vi "Init Channels.vi"(8 "error in (no error)":errorcluster, 11 "Device Item Ref In":T2 format="%.0x") -> (0 "error out":errorcluster, 1 "Output Refs":T1[](array[typedef]) format="%.0x", 2 "Output Values":dbl[](array[numeric]), 3 "Input Refs":T1[](array[typedef]) format="%.0x", 5 "Input Values":dbl[](array[numeric]))   [LabVIEW 2011, in "Interpolate 1D Array Custom Device.lvlib"]
uses:
  Interpolate 1D Array Custom Device.lvlib
  <vilib>/NI Veristand/Custom Device API/Custom Device Item Ref.ctl
  <vilib>/NI Veristand/Custom Device API/Data Reference.ctl
  <vilib>/NI Veristand/Custom Device API/Custom Device Channel Type.ctl
  <vilib>/NI Veristand/Custom Device API/Data Access Type.ctl
  <vilib>/NI Veristand/Custom Device API/Custom Device API.lvlib
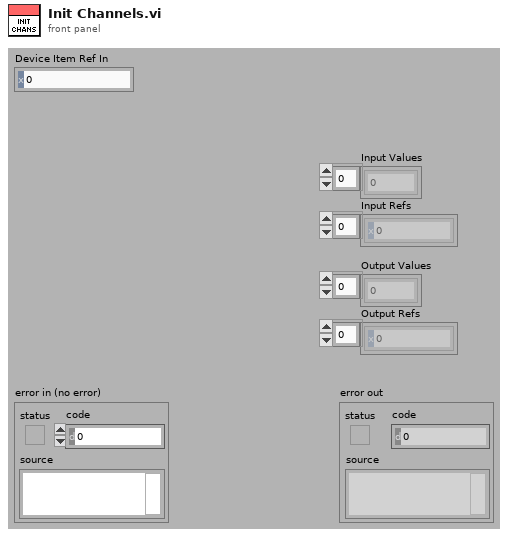
[diagram p1: front panel]
types:
  T1 = typedef "Custom Device API.lvlib/Data Reference.ctl" = i32
  T2 = typedef "Custom Device API.lvlib/Custom Device Item Ref.ctl" = u64
  T3 = typedef "Custom Device API.lvlib/Custom Device Channel Type.ctl" = enum16{"Input", "Output"}
  T4 = typedef "Custom Device API.lvlib/Data Access Type.ctl" = enum16{"Read", "Write"}
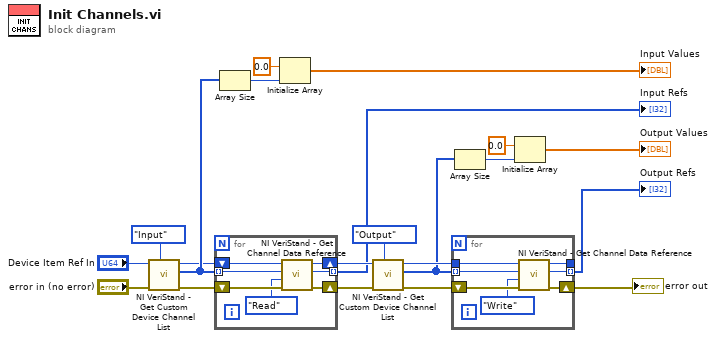
[diagram p0: block diagram]
diagram:
  n1 = call <vilib>:"NI VeriStand - Get Custom Device Channel List.vi"("Channel Type"=Custom_Device_Channel_Type."Input", "error in (no error)"="error in (no error)", "Device Ref in"="Device Item Ref In") -> ("error out"=w12:errorcluster, "Specified Channel Ref List"=w13:T2[], "Device Ref out"=w11:T2)  [unwired: 6 out]
  n2 = for {
    shift-right: [w23] -> w20
    shift-left: w11 -> [w27]
    tunnel: w13 -> [w26] mode=indexing
    shift-right: [w24] -> w16
    shift-left: w12 -> [w28]
    tunnel: [w22] -> w3 mode=indexing
    n3 = call <vilib>:"NI VeriStand - Get Channel Data Reference.vi"("error in (no error)"=w28, "Access"=Data_Access_Type."Read", "Channel Ref in"=w26, "Device Ref in"=w27) -> ("error out"=w24:errorcluster, "Channel Data Reference"=w22:T1, "Device Ref out"=w23:T2)  [unwired: 5 out]
  }
  "Input Refs" <- w3
  n4 = Array Size(array=w13) -> (size(s)=w8:i32)
  n5 = Initialize Array(0.0 ("element"), w8) -> (→"Input Values":dbl[])
  n6 = call <vilib>:"NI VeriStand - Get Custom Device Channel List.vi"("Channel Type"=Custom_Device_Channel_Type."Output", "error in (no error)"=w16, "Device Ref in"=w20) -> ("error out"=w14:errorcluster, "Specified Channel Ref List"=w19:T2[], "Device Ref out"=w21:T2)  [unwired: 6 out]
  n7 = for {
    tunnel: w19 -> [w33] mode=indexing
    shift-right: [w31] -> w5
    shift-left: w14 -> [w35]
    tunnel: [w30] -> w2 mode=indexing
    tunnel: w21 -> [w34]
    tunnel: [w29] -> _
    n8 = call <vilib>:"NI VeriStand - Get Channel Data Reference.vi"("error in (no error)"=w35, "Access"=Data_Access_Type."Write", "Channel Ref in"=w33, "Device Ref in"=w34) -> ("error out"=w31:errorcluster, "Channel Data Reference"=w30:T1, "Device Ref out"=w29:T2)  [unwired: 5 out]
  }
  "error out" <- w5
  "Output Refs" <- w2
  n9 = Array Size(array=w19) -> (size(s)=w18:i32)
  n10 = Initialize Array(0.0 ("element"), w18) -> (→"Output Values":dbl[])
